vi "single fit V3.vi"(6 "main VI path":path, 7 "cursor window: fragment":T2, 8 "pond":cdb[][](array[numeric]), 9 "wave packet":cdb[][](array[numeric]), 10 "omega map parameters":T3={"map method"=enum."less trivial", "2:window factor"=1, "left"=3.0, "right"=3.0, "omega"=3.0, "gamma"=3.0, "theta0"=3.0, "use points"=enum."decimated", "z(inf) method"=enum."median"}, 11 "single fit parameters":T4={"number of 2D grid points"=300, "# of points in pond"=339, "# of points in window"=10919, "decimation threshold"=1, "normalization factor"=0.029014793, "pond scale factor "=3.0, "normalized z"=[], "decimated z"=[], "decimated omega"=[], "omega in window"=[], "z in window"=[], "data center"=3.0+0.0i, "inverse"=[], "linear "=[], "omega around"=[], "phase around center"=[], "fit for phase around senter "=[], "three points"={[], []}}) -> (0 "lorentzian out":T6={"Amplitude"=-1.0311345636926572, "omega(0)"=-1.0311345636926572, "Gamma"=-1.0311345636926572, "phase"=-1.0311345636926572, "Q"=-1.0311345636926572, "Norm  Ampl"=-1.0311345636926572, "z (inf)"=-1.0311345636926572+0.0i, "4corners"={"z (-pi/2)"=-1.0311345636926572+0.5736824521422934i, "z(inf)"=-0.5200164984937075+1.0975277942502903i, "z (pi/2)"=-1.0311345636926572+0.5736824521422934i, "z center"=-0.5136528600391839+0.580046090596817i, "z(0)"=-0.5200164984937075+1.0975277942502903i, "radius"=-1.0311345636926572}} {"Q" format="%#_8f"; "phase" format="%#_6f"; "Gamma" format="%#_8f"; "omega(0)" format="%#_8f"}, 2 "omega map parameters out":T3={"map method"=enum."less trivial", "2:window factor"=1, "left"=3.0, "right"=3.0, "omega"=3.0, "gamma"=3.0, "theta0"=3.0, "use points"=enum."decimated", "z(inf) method"=enum."median"}, 3 "single fit parameters out":T4={"number of 2D grid points"=300, "# of points in pond"=339, "# of points in window"=10919, "decimation threshold"=1, "normalization factor"=0.029014793, "pond scale factor "=3.0, "normalized z"=[], "decimated z"=[], "decimated omega"=[], "omega in window"=[], "z in window"=[], "data center"=3.0+0.0i, "inverse"=[], "linear "=[], "omega around"=[], "phase around center"=[], "fit for phase around senter "=[], "three points"={[], []}}, 4 "complex region out":T5={"max re"=1.1965102077412717, "min re"=-1.8034897922587283, "max im"=1.1920568931854867, "min im"=-1.636084117505164, "delta re"=3.0, "delta im"=2.8281410106906506, "center re"=-0.3034897922587282, "delta  z"=3.0+2.8281410106906506i, "center im"=-0.2220136121598386, "center z"=-0.3034897922587282+2.8281410106906506i, "d im"=0.0, "d re"=0.0, "d z"=0.0+0.0i})   [LabVIEW 2010]
uses:
  lorentzian.ctl
  circle corners.ctl
  complex region.ctl
  single fit parameters.ctl
  omega map parameters.ctl
  <vilib>/Utility/miscctls.llb/LVCursorListTypeDef.ctl
  peak - simple guess at omega.vi
  peak - less simple guess at omega.vi
  peak - fix phase.vi
  peak - fit phase around center.vi
  peak - geometry fit.vi
  find circle corners V3.vi
  peak - phase around center.vi
  peak - linear and inverse maps.vi
  peak - calculate lorentzian.vi
  index from range.vi
  <vilib>/Analysis/baseanly.llb/Mean.vi
  <vilib>/Analysis/baseanly.llb/Median.vi
  <vilib>/Analysis/2dsp.llb/Unwrap Phase.vi
  <vilib>/gmath/interp.llb/Interpolate 1D.vi
  <vilib>/gmath/NumericalOptimization/Nonlinear Curve Fit.vi
  <vilib>/gmath/NumericalOptimization/Nonlinear Curve Fit LM.vi
  <vilib>/Utility/error.llb/Clear Errors.vi
  <vilib>/Analysis/6fits.llb/Linear Fit.vi
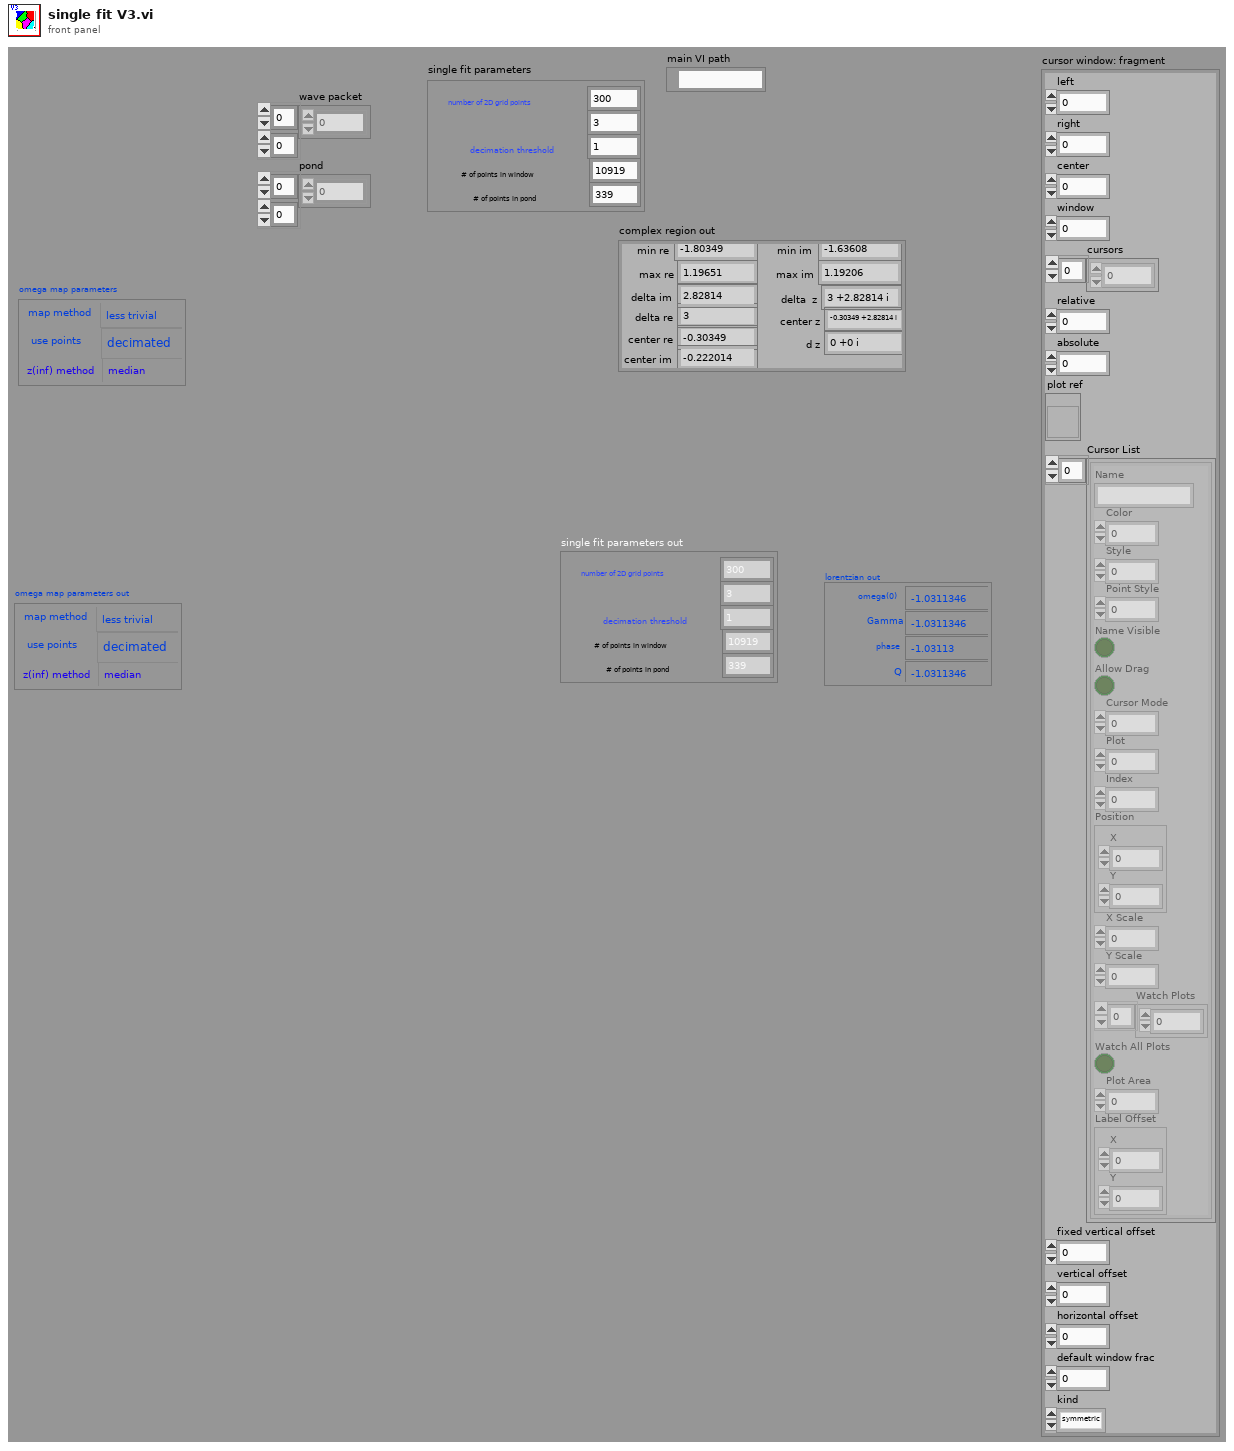
[diagram p1: front panel]
types:
  T1 = typedef "LVCursorListTypeDef.ctl" = cluster{"Name":string, "Color":u32, "Style":u8, "Point Style":u8, "Name Visible":bool, "Allow Drag":bool, "Cursor Mode":u32, "Plot":i32, "Index":i32, "Position":cluster{"X":dbl, "Y":dbl}, "X Scale":u32, "Y Scale":u32, "Watch Plots":i32[], "Watch All Plots":bool, "Plot Area":i32, "Label Offset":cluster{"X":dbl, "Y":dbl}}[]
  T2 = cluster{"left":dbl, "right ":dbl, "center":dbl, "window":dbl, "cursors":i32[], "relative":i32, "absolute":i32, "plot ref":refnum<vi>, "Cursor List":T1, "fixed vertical offset":dbl, "vertical offset":dbl, "horizontal offset":dbl, "default window frac":dbl, "kind":enum16{"symmetric", "skewed", "fancy"}}
  T3 = typedef "omega map parameters.ctl" = cluster{"map method":enum16{"simple", "less trivial", "around center", "geometry"}, "2:window factor":i32, "left":dbl, "right":dbl, "omega":dbl, "gamma":dbl, "theta0":dbl, "use points":enum16{"all in window", "decimated"}, "z(inf) method":enum16{"median", "method 2", "histogram"}}
  T4 = typedef "single fit parameters.ctl" = cluster{"number of 2D grid points":i32, "# of points in pond":i32, "# of points in window":i32, "decimation threshold":i32, "normalization factor":dbl, "pond scale factor ":dbl, "normalized z":cdb[], "decimated z":cdb[], "decimated omega":dbl[], "omega in window":dbl[], "z in window":cdb[], "data center":cdb, "inverse":cdb[], "linear ":cdb[], "omega around":dbl[], "phase around center":dbl[], "fit for phase around senter ":dbl[], "three points":cluster{dbl[], dbl[]}}
  T5 = typedef "complex region.ctl" = cluster{"max re":dbl, "min re":dbl, "max im":dbl, "min im":dbl, "delta re":dbl, "delta im":dbl, "center re":dbl, "delta  z":cdb, "center im":dbl, "center z":cdb, "d im":dbl, "d re":dbl, "d z":cdb}
  T6 = typedef "lorentzian.ctl" = cluster{"Amplitude":dbl, "omega(0)":dbl, "Gamma":dbl, "phase":dbl, "Q":dbl, "Norm  Ampl":dbl, "z (inf)":cdb, "4corners":T7}
  T7 = typedef "circle corners.ctl" = cluster{"z (-pi/2)":cdb, "z(inf)":cdb, "z (pi/2)":cdb, "z center":cdb, "z(0)":cdb, "radius":dbl}
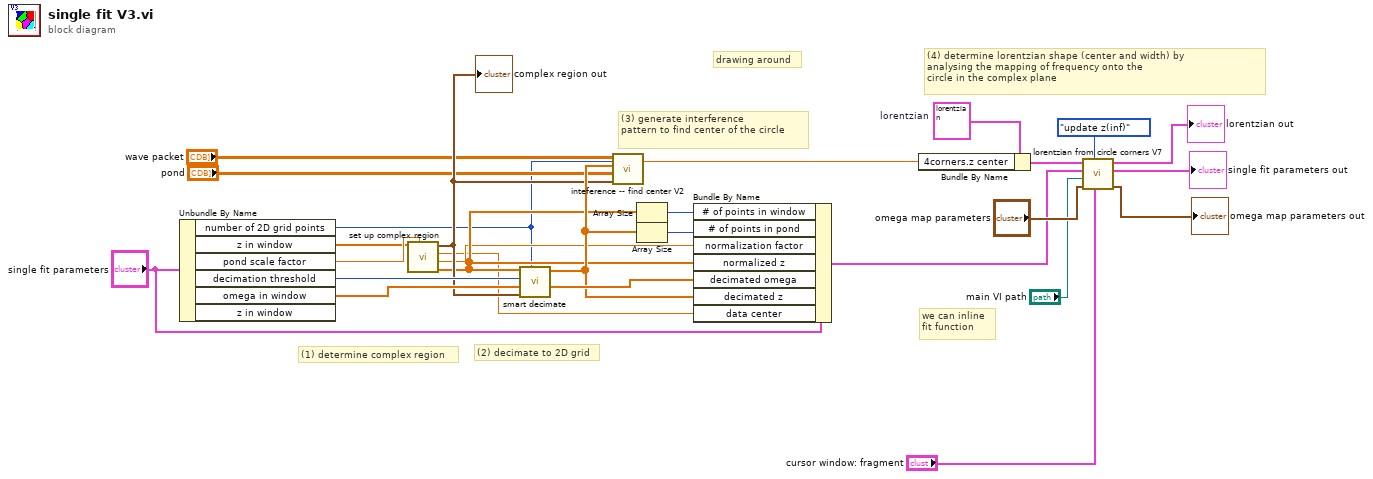
[diagram p0: block diagram]
diagram:
  w6 = T6 {"Amplitude"=-1.0311345636926572, "omega(0)"=-1.0311345636926572, "Gamma"=-1.0311345636926572, "phase"=-1.0311345636926572, "Q"=-1.0311345636926572, "Norm  Ampl"=-1.0311345636926572, "z (inf)"=-1.0311345636926572+0.0i, "4corners"={"z (-pi/2)"=-1.0311345636926572+0.5736824521422934i, "z(inf)"=-0.5200164984937075+1.0975277942502903i, "z (pi/2)"=-1.0311345636926572+0.5736824521422934i, "z center"=-0.5136528600391839+0.580046090596817i, "z(0)"=-0.5200164984937075+1.0975277942502903i, "radius"=-1.0311345636926572}}  # lorentzian
  # "we can inline \nfit function"
  # "(4) determine lorentzian shape (center and width) by \nanalysing the mapping of frequency onto the\ncircle in the complex plane"
  # "(1) determine complex region"
  # "drawing around"
  # "(3) generate interference\npattern to find center of the circle"
  # "(2) decimate to 2D grid"
  n1 = Unbundle By Name("single fit parameters") -> ("number of 2D grid points"=w3:i32, "z in window"=w2:cdb[], "pond scale factor"=w19:dbl, "decimation threshold"=w27:i32, "omega in window"=w22:dbl[])  [unwired: 1 out]
  n2 = call "set up complex region.vi"("scale factor"=w19, "z in window"=w2) -> ("z  normalized"=w17:cdb[], "normalization factor"=w16:dbl, "data center"=w15:cdb, "complex region"=w18:T5)  [unwired: 6 in]
  "complex region out" <- w18
  n3 = call "smart decimate .vi"("number of 2D grid points"=w3, "complex region"=w18, "omega in"=w22, "decimation threshold"=w27, "z in"=w17) -> ("decimated omega"=w24:dbl[], "decimated z"=w21:cdb[])  [unwired: 5 in]
  n4 = call "inteference -- find center V2.vi"("number of points"=w3, "complex region"=w18, "pond"="pond", "point sources"=w21, "wave packet"="wave packet") -> ("z (center)"=w11:cdb)  [unwired: 6 in]
  n5 = Array Size(array=w17) -> (size(s)=w26:i32)
  n6 = Array Size(array=w21) -> (size(s)=w25:i32)
  n7 = Bundle By Name(cluster="single fit parameters", "# of points in window"=w26, "# of points in pond"=w25, "normalization factor"=w16, "normalized z"=w17, "decimated omega"=w24, "decimated z"=w21, "data center"=w15) -> (w12:T4)
  n8 = Bundle By Name(cluster=w6, "4corners.z center"=w11) -> (w5:T6)
  n9 = call "lorentzian from circle corners V7.vi"("cursor window: fragment"="cursor window: fragment", "update z(inf)"=enum16{"update z(inf)", "do not update z(inf)"}."update z(inf)", "omega map rameters in"="omega map parameters", "main VI  path"="main VI path", "parameters in: center detection"=w12, "lorentzian in"=w5) -> ("omega map parameters  out"=→"omega map parameters out":T3, "parameters out  : center detection"=→"single fit parameters out":T4, "lorentzian out"=→"lorentzian out":T6)  [unwired: 3 in]
